vi "Event Handle Loop_Draw_Text.vi"(7 "Active":bool, 8 "error in (no error)":errorcluster, 9 "Text":string, 10 "Picture In":picture, 11 "QMenu Class in":refnum<class "QMenu Class.lvclass">) -> (0 "error out":errorcluster, 2 "Picture Out":picture, 3 "QMenu Class out":refnum<class "QMenu Class.lvclass">)   [LabVIEW 2020, in "QTab.lvlib" / "QMenu Class.lvclass"]
uses:
  QMenu Class.lvclass
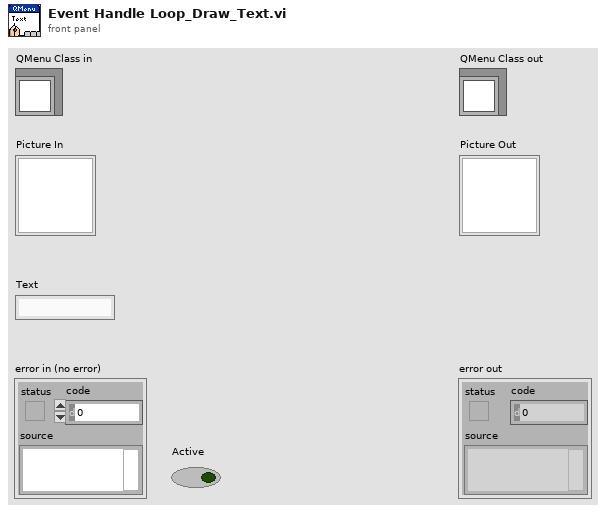
[diagram p1: front panel]
types:
  T1 = cluster{"Font Name:":string, "Size":i16, "Strikeout?":bool, "Italic?":bool, "Underline?":bool, "Outline?":bool, "Shadow?":bool, "Bold?":bool}
  T2 = enum16{"User-specified Font", "Application Font", "System Font", "Dialog Font"}
  T3 = cluster{"horizontal":enum16{"left", "center", "right"}, "vertical":enum16{"top", "center", "bottom"}}
  T4 = typedef "imagedata.ctl" = cluster{"image type":i32, "image depth":i32, "image":u8[], "mask":u8[], "colors":u32[], "Rectangle":cluster{"left":i16, "top":i16, "right":i16, "bottom":i16}}
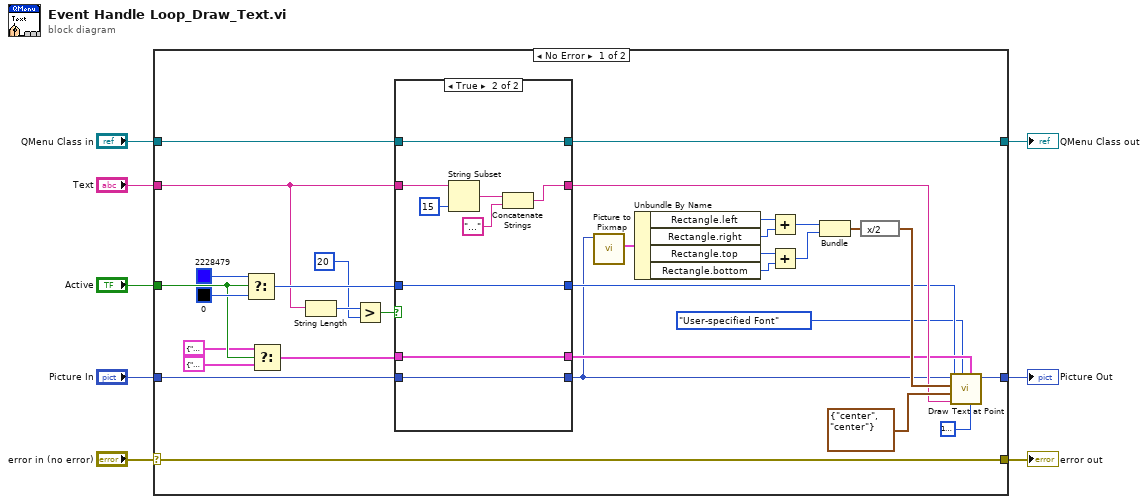
[diagram p0: block diagram]
diagram:
  n1 = case shown="No Error" "error in (no error)" {
    selector: "error in (no error)" -> [w19 w55]
    tunnel: "QMenu Class in" -> [w27 w56]
    tunnel: [w26 w56] -> w7
    tunnel: [w20 _] -> w6
    tunnel: [w19 w55] -> w4
    tunnel: "Picture In" -> [w14 _]
    tunnel: "Text" -> [w11 _]
    tunnel: "Active" -> [w10 _]
    frame No Error {
      n2 = Select(t=u32 2228479 ("color(black)"), s=w10, f=u32 0 ("color(black)")) -> (s? t:f=w25:u32)
      n3 = Select(t=T1 {"Font Name:"="ButtonTab", "Size"=12, "Strikeout?"=FALSE, "Italic?"=FALSE, "Underline?"=TRUE, "Outline?"=FALSE, "Shadow?"=TRUE, "Bold?"=TRUE} ("[user-specified font]"), s=w10, f=T1 {"Font Name:"="ButtonTab", "Size"=12, "Strikeout?"=FALSE, "Italic?"=FALSE, "Underline?"=FALSE, "Outline?"=FALSE, "Shadow?"=FALSE, "Bold?"=FALSE} ("[user-specified font]")) -> (s? t:f=w24:T1)
      n4 = String Length(string=w11) -> (length=w17:i32)
      n5 = Greater?(x=w17, y=20) -> (0:w15:bool)
      n6 = case shown="True" w15 {
        tunnel: w27 -> [w45 w54]
        tunnel: [w45 w54] -> w26
        tunnel: w11 -> [w44 w53]
        tunnel: w25 -> [w43 w48]
        tunnel: w24 -> [w42 w47]
        tunnel: [w44 w49] -> w23
        tunnel: [w43 w48] -> w21
        tunnel: [w42 w47] -> w22
        tunnel: [w41 w46] -> w13
        tunnel: w14 -> [w41 w46]
        frame False {
        }
        frame True {
          n7 = String Subset(string=w53, length (rest)=15 ("length (rest)")) -> (substring=w51:string)  [unwired: 1 in]
          n8 = Concatenate Strings(w51, "..." ("string")) -> (w49:string)
        }
      }
      n9 = call <vilib>:"Picture to Pixmap.vi"("picture"=w13) -> ("image data"=w12:T4)  [unwired: 9 in, 1 out]
      n10 = Unbundle By Name(w12) -> ("Rectangle.left"=w38:i16, "Rectangle.right"=w37:i16, "Rectangle.top"=w36:i16, "Rectangle.bottom"=w35:i16)
      n11 = Add(x=w38, y=w37) -> (x+y=w34:i16)
      n12 = Add(x=w36, y=w35) -> (x+y=w33:i16)
      n13 = Bundle(w34, w33) -> (w32:cluster{i16, i16})  [unwired: 1 in]
      n14 = expression code="x/2"(w32) -> (w31:cluster{i16, i16})
      n15 = call <vilib>:"Draw Text at Point.vi"("BG color(transparent)"=u32 16777216, "[user-specified font]"=w22, "text color(black)"=w21, "desired font(Application)"=T2."User-specified Font", "text"=w23, "alignment(left, top)"=T3 {"horizontal"=enum."center", "vertical"=enum."center"}, "origin"=w31, "picture"=w13) -> ("new picture"=w20:picture)  [unwired: 2 in, 1 out]
    }
    frame Error {
    }
  }
  "error out" <- w4
  "QMenu Class out" <- w7
  "Picture Out" <- w6
